vi "Host-Top-Level.vi"() -> ()   [LabVIEW 2016]
uses:
  <vilib>/rvi/interface/nirviOpenFPGA/nirviOpenFPGA.xnode
  <vilib>/rvi/interface/nirviCloseFPGA/nirviCloseFPGA.xnode
  <vilib>/rvi/interface/nirviMethod/nirviMethod.xnode
  <vilib>/FPGAPlugInAG/Dynamic/niLvFpga_ReadFifo_Dynamic.vi
  <vilib>/rvi/errors/niLvFpgaMergeErrorWithErrorCode.vi
  Fpga/Fpga-Top-Level.vi
  <vilib>/FPGAPlugInAG/Dynamic/niLvFpga_Close_Dynamic.vi
  <vilib>/rvi/interface/RandomDataEmulation/nirviRandomDataOpen.vi
  <vilib>/rvi/interface/common/niFpgaCacheSessionInfoDynamic.vi
panel:
  out "FPGA VI Reference Out":refnum<k20>
  in  "Clear":bool
  out "Data":u32[](array[numeric])
  in  "Read":bool
  in  "error in":errorcluster
  out "Message":string="ERROR!"
  in  "Exit":bool
  in  "Start":bool
  in  "file path (use dialog)":path
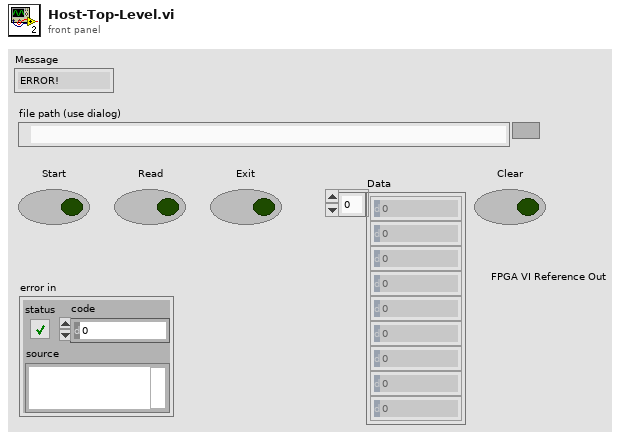
[diagram p1: front panel]
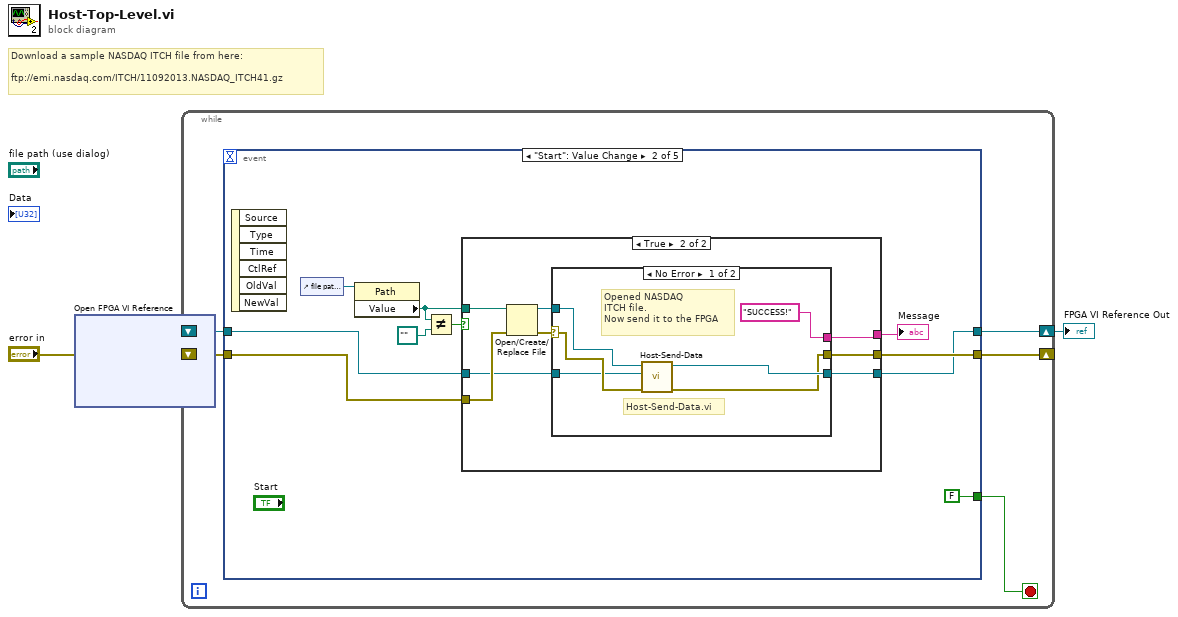
[diagram p0: block diagram]
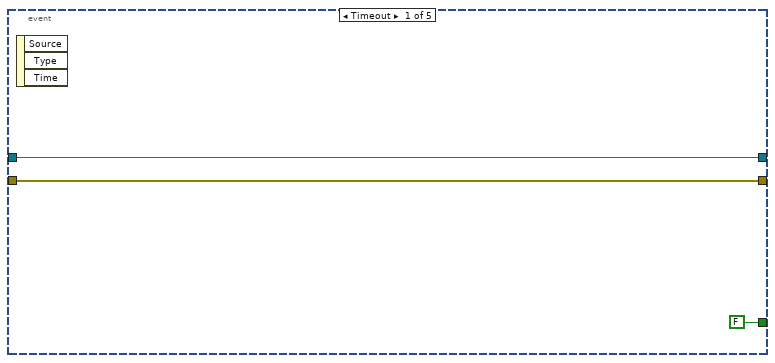
[diagram p2: hidden frame]
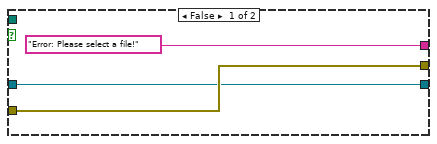
[diagram p3: hidden frame]
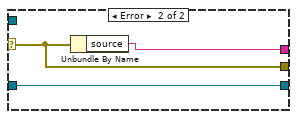
[diagram p4: hidden frame]
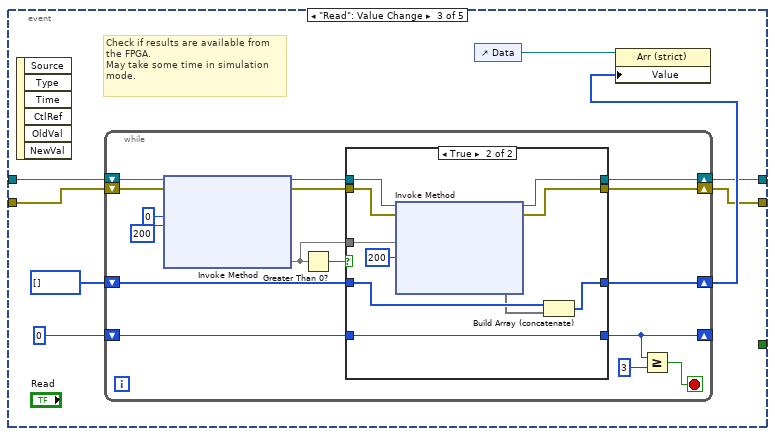
[diagram p5: hidden frame]
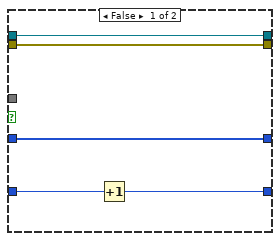
[diagram p6: hidden frame]
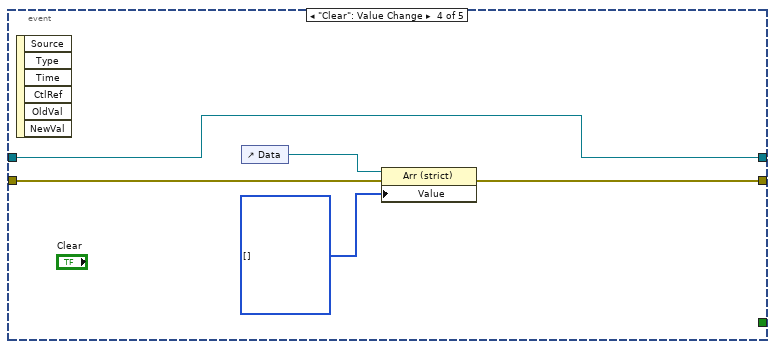
[diagram p7: hidden frame]
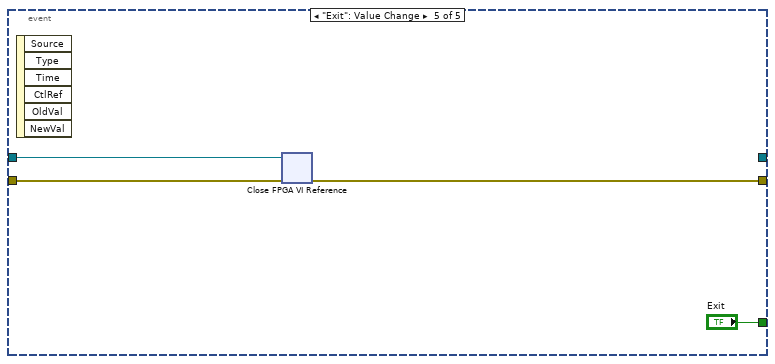
[diagram p8: hidden frame]
diagram:
  # "Download a sample NASDAQ ITCH file from here:\n\nftp://emi.nasdaq.com/ITCH/11092013.NASDAQ_ITCH41.gz"
  n1 = xnode "Open FPGA VI Reference"("error in"="error in") -> ("FPGA VI Reference Out"=w2:refnum<k20>, "error out"=w3:errorcluster)  [unwired: 1 in]
  n2 = while {
    shift-right: [w7] -> _
    shift-left: w3 -> [w8]
    shift-right: [w6] -> w1
    shift-left: w2 -> [w5]
    stop <- w9 stop-if-true
    n3 = event shown="[1] \"Start\": Value Change" {
      selector: _ -> [_ _ _ _ _]
      dyn-events: _ -> [_ _ _ _ _]
      timeout: _ -> [_ _ _ _ _]
      tunnel: [FALSE ("Exit") FALSE ("Exit") _ _ "Exit"] -> w9
      tunnel: w8 -> [w11 w16 w47 w84 w89]
      tunnel: [w11 w14 w43 w83 w88] -> w7
      tunnel: [w10 w13 w44 w82 _] -> w6
      tunnel: w5 -> [w10 w15 w49 w82 w87]
      event Timeout {
        n4 = event-data() -> ()  [unwired: 1 in, 3 out]
      }
      event "Start": Value Change {
        n5 = event-data() -> ()  [unwired: 1 in, 6 out]
        n6 = control-ref of="file path (use dialog)"() -> (w21:refnum<vi>)
        n7 = property class="Path"(reference=w21) -> ("Value"=w20:path)  [unwired: 1 in, 2 out]
        n8 = Not Equal?(x=w20, y=path "" ("Value")) -> (x != y?=w18:bool)
        n9 = case shown="True" w18 {
          tunnel: w20 -> [_ w33]
          tunnel: ["Error: Please select a file!" w30] -> w17
          tunnel: w16 -> [w24 w32]
          tunnel: w15 -> [w23 w29]
          tunnel: [w24 w28] -> w14
          tunnel: [w23 w27] -> w13
          frame False {
          }
          frame True {
            n10 = Open/Create/Replace File(file path (use dialog)=w33, error in=w32) -> (refnum out=w26:refnum<file>, error out=w31:errorcluster)  [unwired: 4 in, 1 out]
            n11 = case shown="No Error" w31 {
              selector: w31 -> [w37 w40]
              tunnel: ["SUCCESS!" w42] -> w30
              tunnel: w29 -> [w34 w41]
              tunnel: [w35 w40] -> w28
              tunnel: [w38 w41] -> w27
              tunnel: w26 -> [w36 _]
              frame No Error {
                # "Host-Send-Data.vi"
                # "Opened NASDAQ\nITCH file.\nNow send it to the FPGA"
                n12 = call "Host-Send-Data.vi"("error in\n(no error)"=w37, "FPGA VI Reference In"=w34, "Byte Stream\nFile in"=w36) -> ("error out"=w35:errorcluster, "FPGA VI Reference Out"=w38:refnum<k20>)  [unwired: 7 in]
              }
              frame Error {
                n13 = Unbundle By Name(w40) -> ("source"=w42:string)
              }
            }
          }
        }
        "Message" <- w17
      }
      event "Read": Value Change {
        # "Check if results are available from\nthe FPGA.\nMay take some time in simulation\nmode."
        n14 = event-data() -> ()  [unwired: 1 in, 6 out]
        n15 = while {
          shift-right: [w55] -> w45
          shift-left: u32[] [] ("Data 2") -> [w56]
          shift-right: [w58] -> w44
          shift-left: w49 -> [w66]
          shift-right: [w57] -> w43
          shift-left: w47 -> [w59]
          shift-right: [w53] -> _
          shift-left: 0 -> [w54]
          stop <- w51 stop-if-true
          n16 = xnode "Invoke Method"("FPGA VI Reference In"=w66, "error in"=w59, "Number of Elements"=u32 0, "Timeout (ms)"=200) -> ("FPGA VI Reference Out"=w61:refnum<k20>, "error out"=w60:errorcluster, "Elements Remaining"=w62)  [unwired: 1 out]
          n17 = Greater Than 0?(x=w62) -> (x > 0?=w63:bool)
          n18 = case shown="True" w63 {
            tunnel: w62 -> [_ w81]
            tunnel: w61 -> [w71 w79]
            tunnel: w60 -> [w70 w78]
            tunnel: [w71 w77] -> w58
            tunnel: [w70 w76] -> w57
            tunnel: w56 -> [w69 w75]
            tunnel: [w69 w73] -> w55
            tunnel: [w67 w72] -> w53
            tunnel: w54 -> [w68 w72]
            frame False {
              n19 = Increment(x=w68) -> (x+1=w67:i32)
            }
            frame True {
              n20 = xnode "Invoke Method"("FPGA VI Reference In"=w79, "error in"=w78, "Number of Elements"=w81, "Timeout (ms)"=200) -> ("FPGA VI Reference Out"=w77:refnum<k20>, "error out"=w76:errorcluster, "Data"=w74:void[])  [unwired: 1 out]
              n21 = Build Array (concatenate)(w75, w74) -> (w73:u32[])
            }
          }
          n22 = Greater Or Equal?(x=w53, y=3) -> (x >= y?=w51:bool)
        }
        n23 = control-ref of="Data"() -> (w50:refnum<vi>)
        n24 = property class="Arr (strict)"(reference=w50, "Value"=w45) -> ()  [unwired: 1 in, 2 out]
      }
      event "Clear": Value Change {
        n25 = event-data() -> ()  [unwired: 1 in, 6 out]
        n26 = control-ref of="Data"() -> (w85:refnum<vi>)
        n27 = property class="Arr (strict)"(reference=w85, error in=w84, "Value"=u32[] []) -> (error out=w83:errorcluster)  [unwired: 1 out]
      }
      event "Exit": Value Change {
        n28 = event-data() -> ()  [unwired: 1 in, 6 out]
        n29 = xnode "Close FPGA VI Reference"("FPGA VI Reference In"=w87, "error in"=w89) -> ("error out"=w88:errorcluster)
      }
    }
  }
  "FPGA VI Reference Out" <- w1
